vi "Configure Pin.vi"(7 "Polarity (0: Positive)":i32(ring) items=["Positive", "Negative"], 8 "error in (no error)":errorcluster {"code" format="%.0x"}, 9 "Pin Function (0: Digital Input/Output)":i32(ring) items=["Digital Input/Output", "Digital Input-only", "Trigger Output", "Trigger Input", "Fault", "Inhibit", "ON Couple", "OFF Couple"], 10 "Pin Name (0: Pin 1)":u16(ring) items=["Pin 1", "Pin 2", "Pin 3", "Pin 4", "Pin 5", "Pin 6", "Pin 7"], 11 "VISA resource name":refnum<visa-resource-name>) -> (0 "error out":errorcluster {"code" format="%.0x"}, 3 "VISA resource name out":refnum<visa-resource-name>)   [LabVIEW 2016, in "Agilent N6700 Series.lvlib"]
doc: "Configures digital port pin functions and polarity."
uses:
  <instrlib>/Agilent N6700 Series/Agilent N6700 Series.lvlib
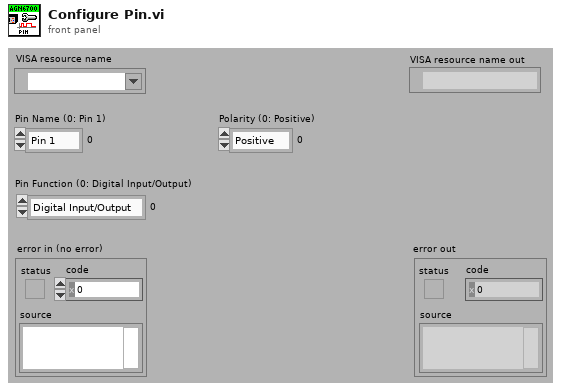
[diagram p1: front panel]
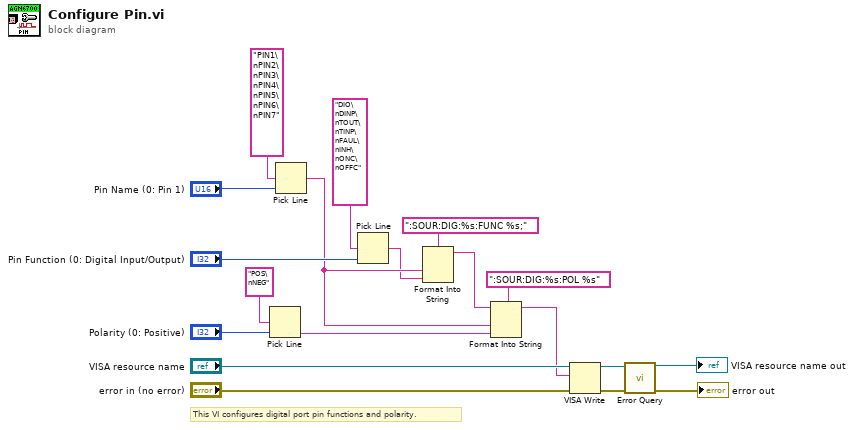
[diagram p0: block diagram]
diagram:
  # "This VI configures digital port pin functions and polarity."
  n1 = Pick Line(multi-line string="POS\nNEG", line index="Polarity (0: Positive)") -> (output string=w10:string)  [unwired: 1 in]
  n2 = Pick Line(multi-line string="PIN1\nPIN2\nPIN3\nPIN4\nPIN5\nPIN6\nPIN7", line index="Pin Name (0: Pin 1)") -> (output string=w9:string)  [unwired: 1 in]
  n3 = Pick Line(multi-line string="DIO\nDINP\nTOUT\nTINP\nFAUL\nINH\nONC\nOFFC", line index="Pin Function (0: Digital Input/Output)") -> (output string=w8:string)  [unwired: 1 in]
  n4 = Format Into String(format string=":SOUR:DIG:%s:FUNC %s;", w9, w8) -> (resulting string=w7:string)  [unwired: 2 in, 1 out]
  n5 = Format Into String(format string=":SOUR:DIG:%s:POL %s", initial string=w7, w9, w10) -> (resulting string=w5:string)  [unwired: 1 in, 1 out]
  n6 = VISA Write(VISA resource name="VISA resource name", write buffer=w5, error in (no error)="error in (no error)") -> (VISA resource name out=w2:refnum<visa-resource-name>, error out=w1:errorcluster)  [unwired: 1 out]
  n7 = call <instrlib>:"Error Query.vi"("VISA resource name"=w2, "error in (no error)"=w1) -> ("VISA resource name out"=→"VISA resource name out":refnum<visa-resource-name>, "error out"=→"error out":errorcluster)  [unwired: 10 in, 2 out]
